vi "9201 8Ch Analog Input.vi"(1 "9201 I/O":T1={"9201 AI0"="NI 9201/AI0", "9201 AI1"="NI 9201/AI1", "9201 AI2"="NI 9201/AI2", "9201 AI3"="NI 9201/AI3", "9201 AI4"="NI 9201/AI4", "9201 AI5"="NI 9201/AI5", "9201 AI6"="NI 9201/AI6", "9201 AI7"="NI 9201/AI7"}) -> (0 "Packets":u64[](array[numeric]))   [LabVIEW 2010]
uses:
  <vilib>/eio/EIONode/EIONode.xnode
  <vilib>/rvi/eio/nirviEIOImplementation/nirviEIOImplementation.xnode
  <vilib>/rvi/eio/common/nirviEmuClasses.ctl
  <vilib>/rvi/eio/common/nirviEmuTemplateMethod_noerrors.vi
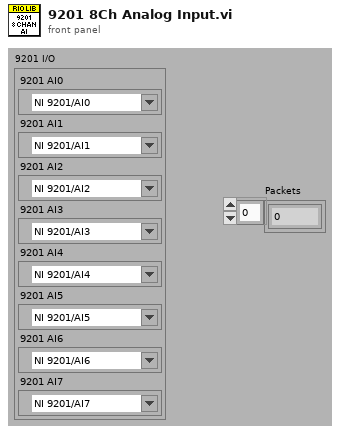
[diagram p1: front panel]
types:
  T1 = cluster{"9201 AI0":refnum<k21>, "9201 AI1":refnum<k21>, "9201 AI2":refnum<k21>, "9201 AI3":refnum<k21>, "9201 AI4":refnum<k21>, "9201 AI5":refnum<k21>, "9201 AI6":refnum<k21>, "9201 AI7":refnum<k21>}
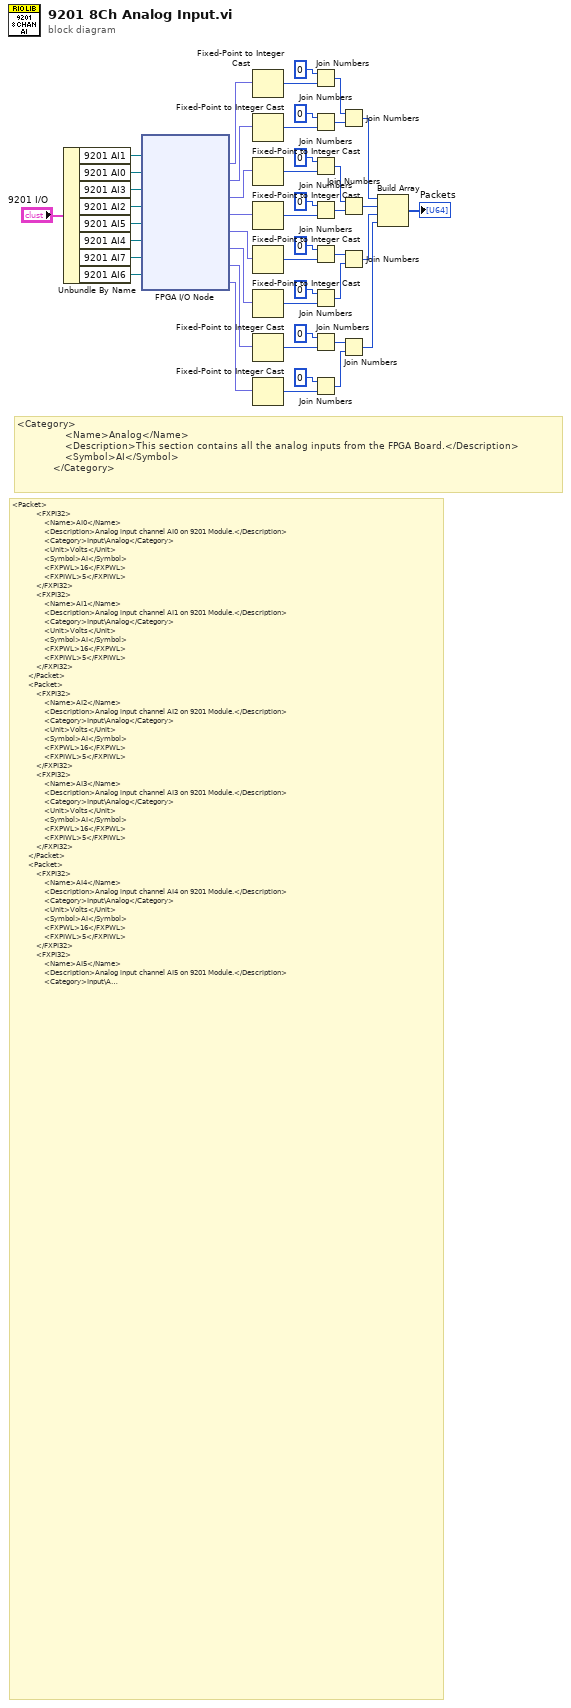
[diagram p0: block diagram]
diagram:
  # "<Category>\n                <Name>Analog</Name>\n                <Description>This section contains all the analog inputs from the FPGA Board.</Description>\n                <Symbol>AI</Symbol>\n            </Category>"
  # "<Packet>\n            <FXPI32>\n                <Name>AI0</Name>\n                <Description>Analog input channel AI0 on 9201 Module.</Description>\n                <Category>Input\\Analog</Category>\n                <Unit>Volts</Unit>\n                <Symbol>AI</Symbol>\n                <FXPWL>16</FXPWL>\n                <FXPIWL>5</FXPIWL>\n            </FXPI32>\n            <FXPI32>\n                <Name>AI1</Name>\n                <Description>Analog input channel AI1 on 9201 Module.</Description>\n                <Category>Input\\Analog</Category>\n                <Unit>Volts</Unit>\n                <Symbol>AI</Symbol>\n                <FXPWL>16</FXPWL>\n                <FXPIWL>5</FXPIWL>\n            </FXPI32>\n        </Packet>\n        <Packet>\n            <FXPI32>\n                <Name>AI2</Name>\n                <Description>Analog input channel AI2 on 9201 Module.</Description>\n                <Category>Input\\Analog</Category>\n                <Unit>Volts</Unit>\n                <Symbol>AI</Symbol>\n                <FXPWL>16</FXPWL>\n                <FXPIWL>5</FXPIWL>\n            </FXPI32>\n            <FXPI32>\n                <Name>AI3</Name>\n                <Description>Analog input channel AI3 on 9201 Module.</Description>\n                <Category>Input\\Analog</Category>\n                <Unit>Volts</Unit>\n                <Symbol>AI</Symbol>\n                <FXPWL>16</FXPWL>\n                <FXPIWL>5</FXPIWL>\n            </FXPI32>\n        </Packet>\n        <Packet>\n            <FXPI32>\n                <Name>AI4</Name>\n                <Description>Analog input channel AI4 on 9201 Module.</Description>\n                <Category>Input\\Analog</Category>\n                <Unit>Volts</Unit>\n                <Symbol>AI</Symbol>\n                <FXPWL>16</FXPWL>\n                <FXPIWL>5</FXPIWL>\n            </FXPI32>\n            <FXPI32>\n                <Name>AI5</Name>\n                <Description>Analog input channel AI5 on 9201 Module.</Description>\n                <Category>Input\\Analog</Category>\n                <Unit>Volts</Unit>\n                <Symbol>AI</Symbol>\n                <FXPWL>16</FXPWL>\n                <FXPIWL>5</FXPIWL>\n            </FXPI32>\n        </Packet>\n        <Packet>\n            <FXPI32>\n                <Name>AI6</Name>\n                <Description>Analog input channel AI6 on 9201 Module.</Description>\n                <Category>Input\\Analog</Category>\n                <Unit>Volts</Unit>\n                <Symbol>AI</Symbol>\n                <FXPWL>16</FXPWL>\n                <FXPIWL>5</FXPIWL>\n            </FXPI32>\n            <FXPI32>\n                <Name>AI7</Name>\n                <Description>Analog input channel AI7 on 9201 Module.</Description>\n                <Category>Input\\Analog</Category>\n                <Unit>Volts</Unit>\n                <Symbol>AI</Symbol>\n                <FXPWL>16</FXPWL>\n                <FXPIWL>5</FXPIWL>\n            </FXPI32>\n        </Packet>"
  n1 = Unbundle By Name("9201 I/O") -> ("9201 AI1"=w42:refnum<k21>, "9201 AI0"=w44:refnum<k21>, "9201 AI3"=w43:refnum<k21>, "9201 AI2"=w45:refnum<k21>, "9201 AI5"=w38:refnum<k21>, "9201 AI4"=w39:refnum<k21>, "9201 AI7"=w40:refnum<k21>, "9201 AI6"=w41:refnum<k21>)
  n2 = xnode "FPGA I/O Node"("FPGA I/O In"=w42, "FPGA I/O In"=w44, "FPGA I/O In"=w43, "FPGA I/O In"=w45, "FPGA I/O In"=w38, "FPGA I/O In"=w39, "FPGA I/O In"=w40, "FPGA I/O In"=w41) -> ("I/O Item"=w35:fxp<+/-,16,5>, "I/O Item"=w30:fxp<+/-,16,5>, "I/O Item"=w23:fxp<+/-,16,5>, "I/O Item"=w22:fxp<+/-,16,5>, "I/O Item"=w16:fxp<+/-,16,5>, "I/O Item"=w13:fxp<+/-,16,5>, "I/O Item"=w3:fxp<+/-,16,5>, "I/O Item"=w2:fxp<+/-,16,5>)  [unwired: 8 out]
  n3 = Fixed-Point to Integer Cast(1:w35) -> (0:w34:i16)
  n4 = Fixed-Point to Integer Cast(1:w30) -> (0:w31:i16)
  n5 = Fixed-Point to Integer Cast(1:w23) -> (0:w27:i16)
  n6 = Fixed-Point to Integer Cast(1:w22) -> (0:w24:i16)
  n7 = Fixed-Point to Integer Cast(1:w16) -> (0:w18:i16)
  n8 = Fixed-Point to Integer Cast(1:w13) -> (0:w14:i16)
  n9 = Fixed-Point to Integer Cast(1:w3) -> (0:w4:i16)
  n10 = Fixed-Point to Integer Cast(1:w2) -> (0:w7:i16)
  n11 = Join Numbers(hi=i16 0, lo=w34) -> ((hi.lo)=w29:u32)
  n12 = Join Numbers(hi=i16 0, lo=w31) -> ((hi.lo)=w28:u32)
  n13 = Join Numbers(hi=i16 0, lo=w27) -> ((hi.lo)=w21:u32)
  n14 = Join Numbers(hi=i16 0, lo=w24) -> ((hi.lo)=w20:u32)
  n15 = Join Numbers(hi=i16 0, lo=w18) -> ((hi.lo)=w12:u32)
  n16 = Join Numbers(hi=i16 0, lo=w14) -> ((hi.lo)=w11:u32)
  n17 = Join Numbers(hi=i16 0, lo=w4) -> ((hi.lo)=w8:u32)
  n18 = Join Numbers(hi=i16 0, lo=w7) -> ((hi.lo)=w9:u32)
  n19 = Join Numbers(hi=w29, lo=w28) -> ((hi.lo)=w37:u64)
  n20 = Join Numbers(hi=w21, lo=w20) -> ((hi.lo)=w19:u64)
  n21 = Join Numbers(hi=w12, lo=w11) -> ((hi.lo)=w10:u64)
  n22 = Join Numbers(hi=w8, lo=w9) -> ((hi.lo)=w1:u64)
  n23 = Build Array(w37, w19, w10, w1) -> (→"Packets":u64[])
